vi "Vis-Element zeichnen.vi"(6 "Editor-Farbe":u32, 7 "Aktion":T1, 8 "Wert-String":string, 9 "Schritt":T2={"Schritt-Typ"=enum."leer", "Schritt-Daten"=variant(string "dummy")}, 11 "Bild alt":picture) -> (3 "Bild neu":picture)   [LabVIEW 2020, in "Anlagenuebersicht.lvlib" / "VisBx Anzeige.lvlib"]
doc: "Zeichnet das Bildelement einer Visualisierung, das in \"Schritt\" in Form eines Clusters aus Schritt-Typ (zB. Linie, Rechteck,..) und zugehörigen Parametern (Variant Schrittdaten) übergeben wird.\nFür Ziffernanzeigen oder variablen Text wird in \"Wert-String\" der darzustellende Inhalt übernommen. \n\nDie Eingangsparameter \"Aktion\" und \"Editor-Farbe\" werden in der Visualiserung \"VisBx-Anzeige\" nicht gebraucht.\n\nAktion (Enum): \nStandardwert \"Bewegtbild\" (zeichnet zB. Ziffernanzeige mit variablem Text).\n\"Fixbild\" (zeichnet zB. Ziffernanzeige mit festem Text aus Schrittdaten).\n\"Suchbild\" (zeichnet Elemente mit \"Editor-Farbe\", die beim Editieren eine Zuordnung eines Pixels zu einem Zeichenelement im Speicher ermöglicht)."
uses:
  VisBx Anzeige.lvlib
  VisParameter/VisSchritt.ctl
  VisParameter/VisSchritt-Typ.ctl
  Vis-Element zeichnen Aktion.ctl
  VisParameter/Param Punkt.ctl
  VisParameter/VisPunkt.ctl
  VisParameter/VisStift.ctl
  VisParameter/Param Linie.ctl
  VisParameter/Param Linienzug.ctl
  VisParameter/Param Text.ctl
  VisParameter/Param Ziffernanzeige.ctl
  VisParameter/Param Rechteck.ctl
  VisParameter/VisRechteck.ctl
  VisParameter/Param Rechteck rund.ctl
  VisParameter/Param Ellipse.ctl
  VisParameter/Param Bogen.ctl
  VisParameter/Param Kreis.ctl
  VisParameter/Param Pixmap.ctl
  <vilib>/picture/picture.llb/Draw True-Color Pixmap.vi
  VisParameter/VisParam-Typdef.lvlib
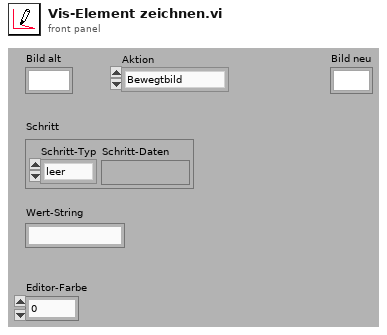
[diagram p1: front panel]
types:
  T1 = typedef "Anlagenuebersicht.lvlib/VisBx Anzeige.lvlib/Vis-Element zeichnen Aktion.ctl" = enum16{"Bewegtbild", "Fixbild", "Suchbild"}
  T2 = typedef "VisParam-Typdef.lvlib/VisSchritt.ctl" = cluster{"Schritt-Typ":T3, "Schritt-Daten":variant}
  T3 = typedef "VisParam-Typdef.lvlib/VisSchritt-Typ.ctl" = enum16{"leer", "Punkt", "Linie", "Linienzug", "Fixtext", "Textrechteck", "Ziffernanzeige", "Rechteck", "Rechteck rund", "Ellipse", "Bogen", "Kreis", "Pixmap"}
  T4 = typedef "VisParam-Typdef.lvlib/Param Punkt.ctl" = cluster{"Punkt":T5, "Farbe":u32, "Stift":T6}
  T5 = typedef "VisParam-Typdef.lvlib/VisPunkt.ctl" = cluster{"x":i16, "y":i16}
  T6 = typedef "VisParam-Typdef.lvlib/VisStift.ctl" = cluster{"Width":u16, "Style":enum32{"Solid", "Dash", "Dot", "DashDot", "DashDotDot"}}
  T7 = typedef "VisParam-Typdef.lvlib/Param Linie.ctl" = cluster{"Startpunkt":T5, "Endpunkt":T5, "Farbe":u32, "Stift":T6}
  T8 = typedef "VisParam-Typdef.lvlib/Param Linienzug.ctl" = cluster{"Endpunkte":T5[], "Farbe":u32, "Füllen":bool, "Stift":T6}
  T9 = typedef "VisParam-Typdef.lvlib/Param Text.ctl" = cluster{"Text":string, "Ursprung":T5, "Schriftgröße":i16, "Farbe":u32, "Ausrichtung":cluster{"horizontal":enum16{"left", "center", "right"}, "vertical":enum16{"top", "center", "bottom"}}}
  T10 = typedef "VisParam-Typdef.lvlib/Param Ziffernanzeige.ctl" = cluster{"Wert-String":string, "Rechteck":cluster{"left":i16, "top":i16, "right":i16, "bottom":i16}, "Schriftgröße":i16, "Textfarbe":u32, "Hintergrund":u32, "Rahmenfarbe":u32}
  T11 = typedef "VisParam-Typdef.lvlib/Param Rechteck.ctl" = cluster{"VisRechteck":T12, "Farbe":u32, "Füllen":bool, "Stift":T6}
  T12 = typedef "VisParam-Typdef.lvlib/VisRechteck.ctl" = cluster{"left":i16, "top":i16, "right":i16, "bottom":i16}
  T13 = cluster{"left":i16, "top":i16, "right":i16, "bottom":i16}
  T14 = typedef "VisParam-Typdef.lvlib/Param Rechteck rund.ctl" = cluster{"VisRechteck":T12, "Farbe":u32, "Füllen":bool, "Rundung":i16, "Stift":T6}
  T15 = typedef "VisParam-Typdef.lvlib/Param Ellipse.ctl" = cluster{"VisRechteck":T12, "Farbe":u32, "Füllen":bool, "Stift":T6}
  T16 = typedef "VisParam-Typdef.lvlib/Param Bogen.ctl" = cluster{"VisRechteck":T12, "Startwinkel":i16, "Winkel":i16, "Farbe":u32, "Füllen":bool, "Stift":T6}
  T17 = typedef "VisParam-Typdef.lvlib/Param Kreis.ctl" = cluster{"Mittelpunkt":T5, "Radius":i16, "Startwinkel":i16, "Winkel":i16, "Farbe":u32, "Füllen":bool, "Stift":T6}
  T18 = typedef "VisParam-Typdef.lvlib/Param Pixmap.ctl" = cluster{"Ecke links oben":T5, "Pixel-Daten":u32[][]}
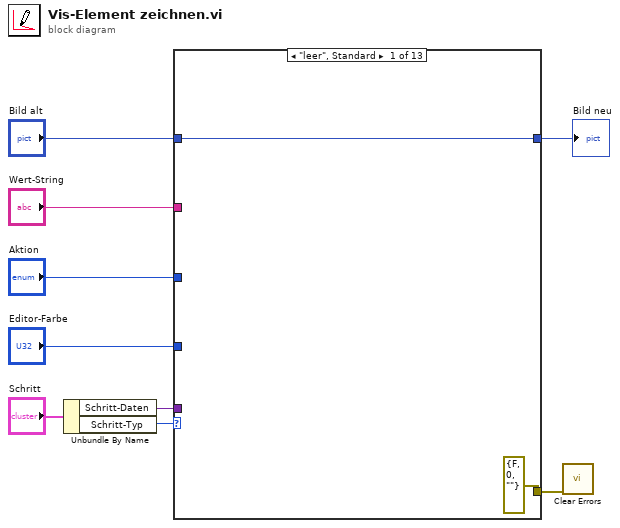
[diagram p0: block diagram]
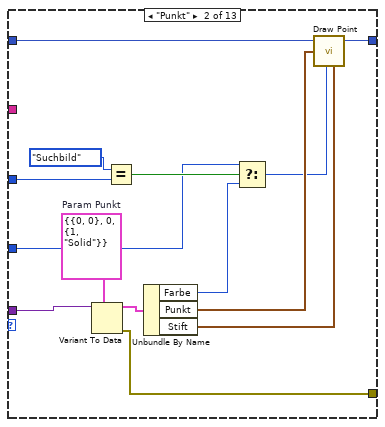
[diagram p2: hidden frame]
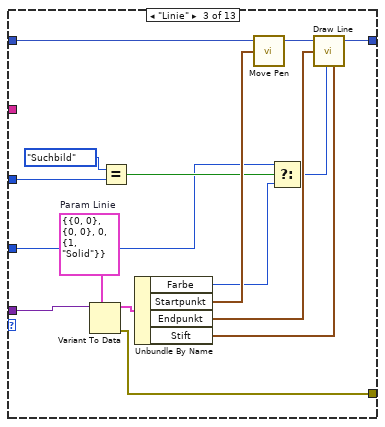
[diagram p3: hidden frame]
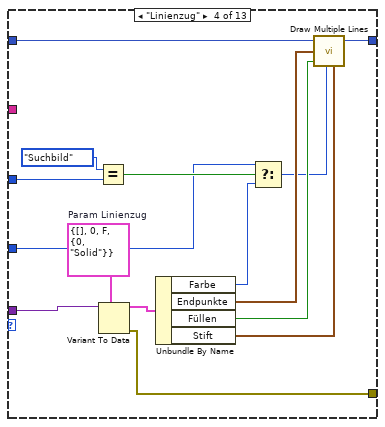
[diagram p4: hidden frame]
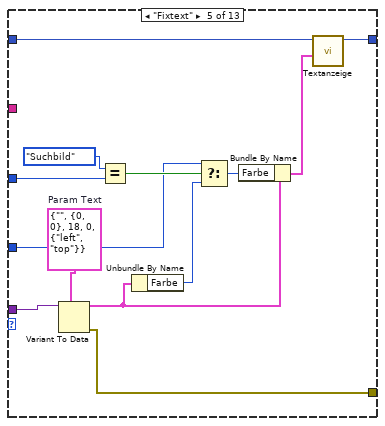
[diagram p5: hidden frame]
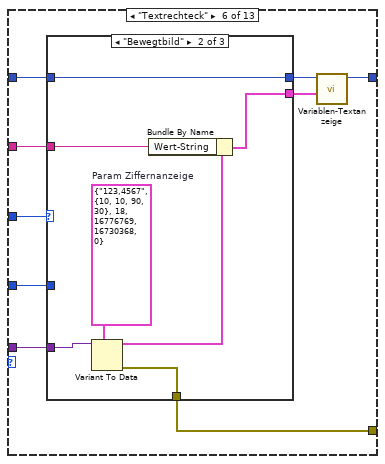
[diagram p6: hidden frame]
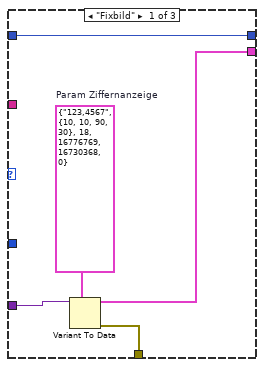
[diagram p7: hidden frame]
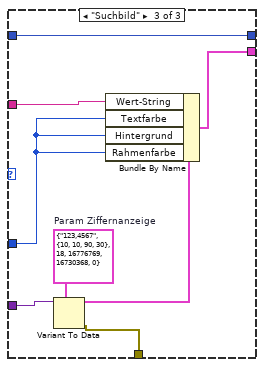
[diagram p8: hidden frame]
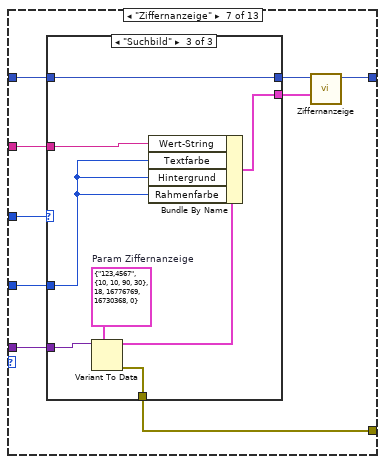
[diagram p9: hidden frame]
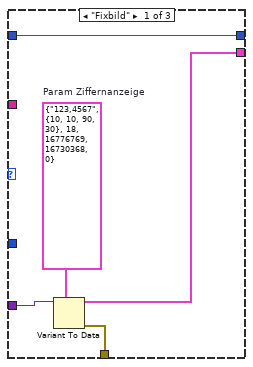
[diagram p10: hidden frame]
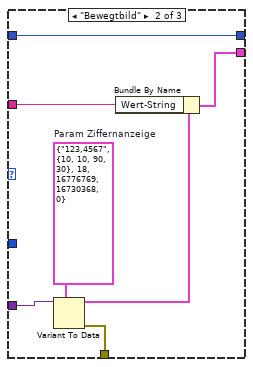
[diagram p11: hidden frame]
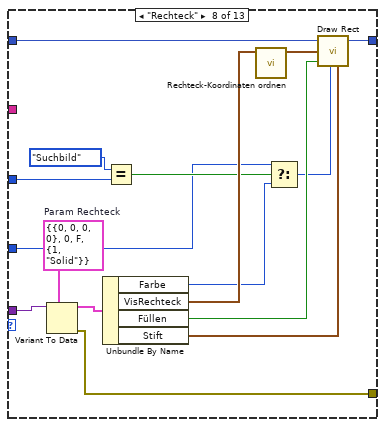
[diagram p12: hidden frame]
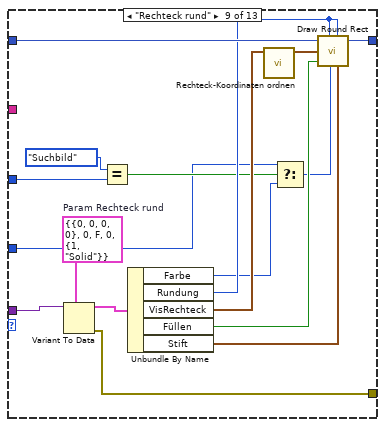
[diagram p13: hidden frame]
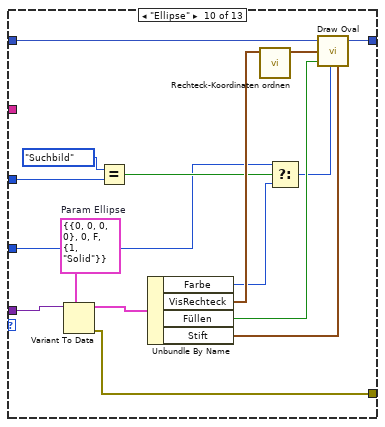
[diagram p14: hidden frame]
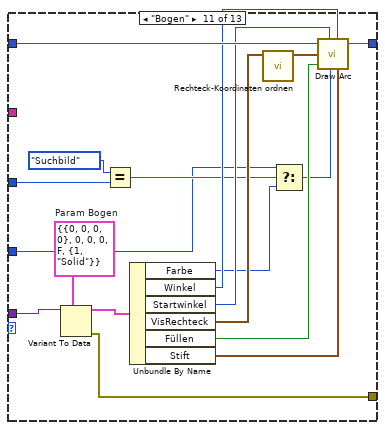
[diagram p15: hidden frame]
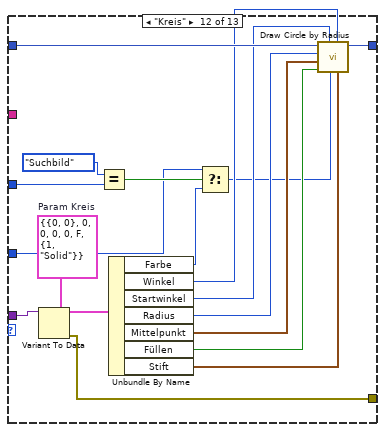
[diagram p16: hidden frame]
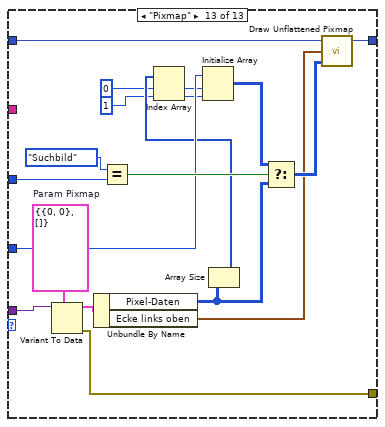
[diagram p17: hidden frame]
diagram:
  n1 = Unbundle By Name("Schritt") -> ("Schritt-Daten"=w9:variant, "Schritt-Typ"=w6:T3)
  n2 = case shown="\"leer\", Standard" w6 {
    tunnel: "Bild alt" -> [w11 w25 w38 w49 w69 w78 w107 w139 w157 w173 w191 w209 w231]
    tunnel: [w11 w24 w41 w56 w68 w74 w102 w140 w158 w174 w192 w210 w230] -> w8
    tunnel: w9 -> [_ w22 w40 w55 w67 w77 w106 w143 w160 w176 w194 w212 w229]
    tunnel: "Wert-String" -> [_ _ _ _ _ w75 w104 _ _ _ _ _ _]
    tunnel: "Aktion" -> [_ w18 w30 w46 w63 w76 w105 w132 w148 w165 w181 w199 w224]
    tunnel: "Editor-Farbe" -> [_ w13 w27 w45 w58 w71 w100 w129 w145 w162 w178 w196 w222]
    tunnel: [errorcluster {"status"=FALSE, "code"=0, "source"=""} ("error out") w12 w26 w42 w57 w70 w99 w128 w144 w161 w177 w195 w213] -> w1
    frame "leer", Default {
    }
    frame "Punkt" {
      w23 = T4 {"Punkt"={"x"=0, "y"=0}, "Farbe"=0, "Stift"={"Width"=1, "Style"=enum."Solid"}}  # Param Punkt
      n3 = Variant To Data(type=w23, Variant=w22) -> (data=w21:T4, error out=w12:errorcluster)  [unwired: 1 in]
      n4 = Equal?(x=Vis-Element_zeichnen_Aktion."Suchbild", y=w18) -> (x = y?=w16:bool)
      n5 = Unbundle By Name(w21) -> ("Farbe"=w14:u32, "Punkt"=w20:T5, "Stift"=w19:T6)
      n6 = Select(t=w13, s=w16, f=w14) -> (s? t:f=w15:u32)
      n7 = call <vilib>:"Draw Point.vi"("picture"=w25, "point(x,y)"=w20, "color(black)"=w15, "pen"=w19) -> ("new picture"=w24:picture)  [unwired: 5 out]
    }
    frame "Linie" {
      w36 = T7 {"Startpunkt"={"x"=0, "y"=0}, "Endpunkt"={"x"=0, "y"=0}, "Farbe"=0, "Stift"={"Width"=1, "Style"=enum."Solid"}}  # Param Linie
      n8 = Variant To Data(type=w36, Variant=w40) -> (data=w39:T7, error out=w26:errorcluster)  [unwired: 1 in]
      n9 = Equal?(x=Vis-Element_zeichnen_Aktion."Suchbild", y=w30) -> (x = y?=w31:bool)
      n10 = Unbundle By Name(w39) -> ("Farbe"=w29:u32, "Startpunkt"=w35:T5, "Endpunkt"=w34:T5, "Stift"=w33:T6)
      n11 = call <vilib>:"Move Pen.vi"("new position"=w35, "picture"=w38) -> ("new picture"=w37:picture)  [unwired: 1 in, 2 out]
      n12 = Select(t=w27, s=w31, f=w29) -> (s? t:f=w28:u32)
      n13 = call <vilib>:"Draw Line.vi"("picture"=w37, "end point"=w34, "color(black)"=w28, "pen"=w33) -> ("new picture"=w41:picture)  [unwired: 1 in, 4 out]
    }
    frame "Linienzug" {
      w52 = T8 {"Endpunkte"=[], "Farbe"=0, "Füllen"=FALSE, "Stift"={"Width"=0, "Style"=enum."Solid"}}  # Param Linienzug
      n14 = Equal?(x=Vis-Element_zeichnen_Aktion."Suchbild", y=w46) -> (x = y?=w47:bool)
      n15 = Variant To Data(type=w52, Variant=w55) -> (data=w54:T8, error out=w42:errorcluster)  [unwired: 1 in]
      n16 = Unbundle By Name(w54) -> ("Farbe"=w44:u32, "Endpunkte"=w51:T5[], "Füllen"=w50:bool, "Stift"=w53:T6)
      n17 = Select(t=w45, s=w47, f=w44) -> (s? t:f=w43:u32)
      n18 = call <vilib>:"Draw Multiple Lines.vi"("picture"=w49, "line endpoints"=w51, "fill?(F)"=w50, "color(black)"=w43, "pen"=w53) -> ("new picture"=w56:picture)  [unwired: 4 out]
    }
    frame "Fixtext" {
      w66 = T9 {"Text"="", "Ursprung"={"x"=0, "y"=0}, "Schriftgröße"=18, "Farbe"=0, "Ausrichtung"={"horizontal"=enum."left", "vertical"=enum."top"}}  # Param Text
      n19 = Variant To Data(type=w66, Variant=w67) -> (data=w62:T9, error out=w57:errorcluster)  [unwired: 1 in]
      n20 = Equal?(x=Vis-Element_zeichnen_Aktion."Suchbild", y=w63) -> (x = y?=w64:bool)
      n21 = Unbundle By Name(w62) -> ("Farbe"=w59:u32)
      n22 = Select(t=w58, s=w64, f=w59) -> (s? t:f=w60:u32)
      n23 = Bundle By Name(cluster=w62, "Farbe"=w60) -> (w61:T9)
      n24 = call "Textanzeige.vi"("Param Text"=w61, "Bild"=w69) -> ("Bild neu"=w68:picture)  [unwired: 9 out]
    }
    frame "Textrechteck" {
      n25 = case shown="\"Bewegtbild\"" w76 {
        tunnel: w78 -> [w80 w86 w94]
        tunnel: w77 -> [w82 w89 w97]
        tunnel: w75 -> [_ w87 w95]
        tunnel: [w80 w86 w94] -> w73
        tunnel: [w81 w85 w93] -> w72
        tunnel: w71 -> [_ _ w92]
        tunnel: [w79 w84 w91] -> w70
        frame "Fixbild" {
          w83 = T10 {"Wert-String"="123,4567", "Rechteck"={"left"=10, "top"=10, "right"=90, "bottom"=30}, "Schriftgröße"=18, "Textfarbe"=16776769, "Hintergrund"=16730368, "Rahmenfarbe"=0}  # Param Ziffernanzeige
          n26 = Variant To Data(type=w83, Variant=w82) -> (data=w81:T10, error out=w79:errorcluster)  [unwired: 1 in]
        }
        frame "Bewegtbild" {
          w90 = T10 {"Wert-String"="123,4567", "Rechteck"={"left"=10, "top"=10, "right"=90, "bottom"=30}, "Schriftgröße"=18, "Textfarbe"=16776769, "Hintergrund"=16730368, "Rahmenfarbe"=0}  # Param Ziffernanzeige
          n27 = Variant To Data(type=w90, Variant=w89) -> (data=w88:T10, error out=w84:errorcluster)  [unwired: 1 in]
          n28 = Bundle By Name(cluster=w88, "Wert-String"=w87) -> (w85:T10)
        }
        frame "Suchbild" {
          w98 = T10 {"Wert-String"="123,4567", "Rechteck"={"left"=10, "top"=10, "right"=90, "bottom"=30}, "Schriftgröße"=18, "Textfarbe"=16776769, "Hintergrund"=16730368, "Rahmenfarbe"=0}  # Param Ziffernanzeige
          n29 = Variant To Data(type=w98, Variant=w97) -> (data=w96:T10, error out=w91:errorcluster)  [unwired: 1 in]
          n30 = Bundle By Name(cluster=w96, "Wert-String"=w95, "Textfarbe"=w92, "Hintergrund"=w92, "Rahmenfarbe"=w92) -> (w93:T10)
        }
      }
      n31 = call "Variablen-Textanzeige.vi"("Param Ziffernanzeige"=w72, "Bild"=w73) -> ("Bild neu"=w74:picture)  [unwired: 9 in]
    }
    frame "Ziffernanzeige" {
      n32 = case shown="\"Suchbild\"" w105 {
        tunnel: w107 -> [w109 w115 w123]
        tunnel: [w109 w115 w123] -> w103
        tunnel: w106 -> [w111 w118 w126]
        tunnel: w104 -> [_ w116 w124]
        tunnel: [w110 w114 w122] -> w101
        tunnel: w100 -> [_ _ w121]
        tunnel: [w108 w113 w120] -> w99
        frame "Fixbild" {
          w112 = T10 {"Wert-String"="123,4567", "Rechteck"={"left"=10, "top"=10, "right"=90, "bottom"=30}, "Schriftgröße"=18, "Textfarbe"=16776769, "Hintergrund"=16730368, "Rahmenfarbe"=0}  # Param Ziffernanzeige
          n33 = Variant To Data(type=w112, Variant=w111) -> (data=w110:T10, error out=w108:errorcluster)  [unwired: 1 in]
        }
        frame "Bewegtbild" {
          w119 = T10 {"Wert-String"="123,4567", "Rechteck"={"left"=10, "top"=10, "right"=90, "bottom"=30}, "Schriftgröße"=18, "Textfarbe"=16776769, "Hintergrund"=16730368, "Rahmenfarbe"=0}  # Param Ziffernanzeige
          n34 = Variant To Data(type=w119, Variant=w118) -> (data=w117:T10, error out=w113:errorcluster)  [unwired: 1 in]
          n35 = Bundle By Name(cluster=w117, "Wert-String"=w116) -> (w114:T10)
        }
        frame "Suchbild" {
          w127 = T10 {"Wert-String"="123,4567", "Rechteck"={"left"=10, "top"=10, "right"=90, "bottom"=30}, "Schriftgröße"=18, "Textfarbe"=16776769, "Hintergrund"=16730368, "Rahmenfarbe"=0}  # Param Ziffernanzeige
          n36 = Variant To Data(type=w127, Variant=w126) -> (data=w125:T10, error out=w120:errorcluster)  [unwired: 1 in]
          n37 = Bundle By Name(cluster=w125, "Wert-String"=w124, "Textfarbe"=w121, "Hintergrund"=w121, "Rahmenfarbe"=w121) -> (w122:T10)
        }
      }
      n38 = call "Ziffernanzeige.vi"("Param Ziffernanzeige"=w101, "Bild"=w103) -> ("Bild neu"=w102:picture)  [unwired: 9 out]
    }
    frame "Rechteck" {
      w141 = T11 {"VisRechteck"={"left"=0, "top"=0, "right"=0, "bottom"=0}, "Farbe"=0, "Füllen"=FALSE, "Stift"={"Width"=1, "Style"=enum."Solid"}}  # Param Rechteck
      n39 = Variant To Data(type=w141, Variant=w143) -> (data=w142:T11, error out=w128:errorcluster)  [unwired: 1 in]
      n40 = Unbundle By Name(w142) -> ("Farbe"=w131:u32, "VisRechteck"=w136:T12, "Füllen"=w138:bool, "Stift"=w137:T6)
      n41 = Equal?(x=Vis-Element_zeichnen_Aktion."Suchbild", y=w132) -> (x = y?=w133:bool)
      n42 = call "Rechteck-Koordinaten ordnen.vi"("Rechteck-Koordinaten"=w136) -> ("Koordinaten geordnet"=w135:T13)  [unwired: 6 in]
      n43 = Select(t=w129, s=w133, f=w131) -> (s? t:f=w130:u32)
      n44 = call <vilib>:"Draw Rect.vi"("picture"=w139, "rect"=w135, "fill?(F)"=w138, "color(black)"=w130, "pen"=w137) -> ("new picture"=w140:picture)  [unwired: 4 out]
    }
    frame "Rechteck rund" {
      w154 = T14 {"VisRechteck"={"left"=0, "top"=0, "right"=0, "bottom"=0}, "Farbe"=0, "Füllen"=FALSE, "Rundung"=0, "Stift"={"Width"=1, "Style"=enum."Solid"}}  # Param Rechteck rund
      n45 = Variant To Data(type=w154, Variant=w160) -> (data=w159:T14, error out=w144:errorcluster)  [unwired: 1 in]
      n46 = Equal?(x=Vis-Element_zeichnen_Aktion."Suchbild", y=w148) -> (x = y?=w149:bool)
      n47 = Unbundle By Name(w159) -> ("Farbe"=w147:u32, "Rundung"=w153:i16, "VisRechteck"=w152:T12, "Füllen"=w156:bool, "Stift"=w155:T6)
      n48 = call "Rechteck-Koordinaten ordnen.vi"("Rechteck-Koordinaten"=w152) -> ("Koordinaten geordnet"=w151:T13)  [unwired: 6 in]
      n49 = Select(t=w145, s=w149, f=w147) -> (s? t:f=w146:u32)
      n50 = call <vilib>:"Draw Round Rect.vi"("picture"=w157, "oval width"=w153, "rect"=w151, "fill?(F)"=w156, "color(black)"=w146, "oval height"=w153, "pen"=w155) -> ("new picture"=w158:picture)  [unwired: 2 out]
    }
    frame "Ellipse" {
      w170 = T15 {"VisRechteck"={"left"=0, "top"=0, "right"=0, "bottom"=0}, "Farbe"=0, "Füllen"=FALSE, "Stift"={"Width"=1, "Style"=enum."Solid"}}  # Param Ellipse
      n51 = Variant To Data(type=w170, Variant=w176) -> (data=w175:T15, error out=w161:errorcluster)  [unwired: 1 in]
      n52 = Equal?(x=Vis-Element_zeichnen_Aktion."Suchbild", y=w165) -> (x = y?=w166:bool)
      n53 = Unbundle By Name(w175) -> ("Farbe"=w164:u32, "VisRechteck"=w168:T12, "Füllen"=w172:bool, "Stift"=w171:T6)
      n54 = call "Rechteck-Koordinaten ordnen.vi"("Rechteck-Koordinaten"=w168) -> ("Koordinaten geordnet"=w169:T13)  [unwired: 6 in]
      n55 = Select(t=w162, s=w166, f=w164) -> (s? t:f=w163:u32)
      n56 = call <vilib>:"Draw Oval.vi"("picture"=w173, "rect"=w169, "fill?(F)"=w172, "color(black)"=w163, "pen"=w171) -> ("new picture"=w174:picture)  [unwired: 4 out]
    }
    frame "Bogen" {
      w188 = T16 {"VisRechteck"={"left"=0, "top"=0, "right"=0, "bottom"=0}, "Startwinkel"=0, "Winkel"=0, "Farbe"=0, "Füllen"=FALSE, "Stift"={"Width"=1, "Style"=enum."Solid"}}  # Param Bogen
      n57 = Variant To Data(type=w188, Variant=w194) -> (data=w193:T16, error out=w177:errorcluster)  [unwired: 1 in]
      n58 = Equal?(x=Vis-Element_zeichnen_Aktion."Suchbild", y=w181) -> (x = y?=w182:bool)
      n59 = Unbundle By Name(w193) -> ("Farbe"=w180:u32, "Winkel"=w187:i16, "Startwinkel"=w186:i16, "VisRechteck"=w185:T12, "Füllen"=w190:bool, "Stift"=w189:T6)
      n60 = call "Rechteck-Koordinaten ordnen.vi"("Rechteck-Koordinaten"=w185) -> ("Koordinaten geordnet"=w184:T13)  [unwired: 6 in]
      n61 = Select(t=w178, s=w182, f=w180) -> (s? t:f=w179:u32)
      n62 = call <vilib>:"Draw Arc.vi"("picture"=w191, "start angle[degrees]"=w186, "rect"=w184, "fill?(F)"=w190, "color(black)"=w179, "arc size[degrees]"=w187, "pen"=w189) -> ("new picture"=w192:picture)  [unwired: 2 out]
    }
    frame "Kreis" {
      w203 = T17 {"Mittelpunkt"={"x"=0, "y"=0}, "Radius"=0, "Startwinkel"=0, "Winkel"=0, "Farbe"=0, "Füllen"=FALSE, "Stift"={"Width"=1, "Style"=enum."Solid"}}  # Param Kreis
      n63 = Variant To Data(type=w203, Variant=w212) -> (data=w211:T17, error out=w195:errorcluster)  [unwired: 1 in]
      n64 = Equal?(x=Vis-Element_zeichnen_Aktion."Suchbild", y=w199) -> (x = y?=w200:bool)
      n65 = Unbundle By Name(w211) -> ("Farbe"=w198:u32, "Winkel"=w205:i16, "Startwinkel"=w204:i16, "Radius"=w202:i16, "Mittelpunkt"=w206:T5, "Füllen"=w208:bool, "Stift"=w207:T6)
      n66 = Select(t=w196, s=w200, f=w198) -> (s? t:f=w197:u32)
      n67 = call <vilib>:"Draw Circle by Radius.vi"("pen"=w207, "arc size(360)"=w205, "color(black)"=w197, "start angle(0)"=w204, "fill?(F)"=w208, "pixel center"=w206, "radius"=w202, "picture"=w209) -> ("new picture"=w210:picture)  [unwired: 3 out]
    }
    frame "Pixmap" {
      w227 = T18 {"Ecke links oben"={"x"=0, "y"=0}, "Pixel-Daten"=[]}  # Param Pixmap
      n68 = Variant To Data(type=w227, Variant=w229) -> (data=w228:T18, error out=w213:errorcluster)  [unwired: 1 in]
      n69 = Unbundle By Name(w228) -> ("Pixel-Daten"=w219:u32[][], "Ecke links oben"=w220:T5)
      n70 = Equal?(x=Vis-Element_zeichnen_Aktion."Suchbild", y=w224) -> (x = y?=w225:bool)
      n71 = Array Size(array=w219) -> (size(s)=w216:i32[])
      n72 = Index Array(array=w216, index #1=0 ("Index"), index #2=1 ("Index")) -> (element #1=w218:i32, element #2=w217:i32)
      n73 = Initialize Array(w222, w218, w217) -> (w221:u32[][])
      n74 = Select(t=w221, s=w225, f=w219) -> (s? t:f=w223:u32[][])
      n75 = call-poly <vilib>:"Draw Unflattened Pixmap.vi"("picture"=w231, "top left point(0, 0)"=w220, "data (RGB format)"=w223) -> ("new picture"=w230:picture)  [unwired: 6 in]
    }
  }
  "Bild neu" <- w8
  n76 = call <vilib>:"Clear Errors.vi"("error in (no error)"=w1) -> ()  [unwired: 5 in, 2 out]
